vi "Populate Column Headers.vi"(8 "error in (no error)":errorcluster, 11 "Column Headers":string[](array[string])) -> (0 "error out":errorcluster)   [LabVIEW 2023, in "RFCalAndFixtureCharact.Common.lvlib"]
uses:
  RFCalAndFixtureCharact.Common.lvlib
  Type Definitions/Dictionary Operation.ctl
  <vilib>/Utility/error.llb/Trim Whitespace One-Sided.vi
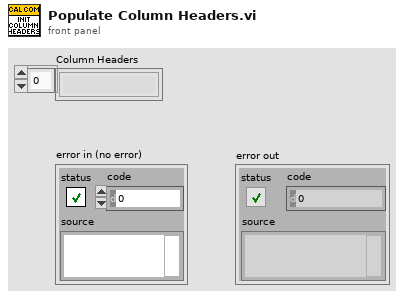
[diagram p1: front panel]
types:
  T1 = typedef "RFCalAndFixtureCharact.Common.lvlib/Dictionary Operation.ctl" = enum16{"Read", "Insert", "Remove", "Clear", "Get All", "Update"}
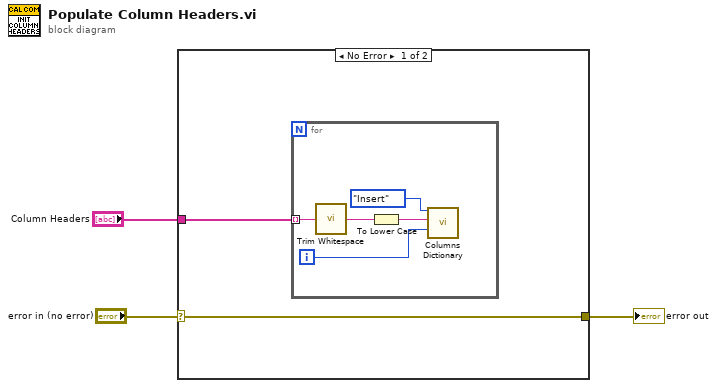
[diagram p0: block diagram]
diagram:
  n1 = case shown="No Error" "error in (no error)" {
    selector: "error in (no error)" -> [w5 w11]
    tunnel: [w5 w11] -> w2
    tunnel: "Column Headers" -> [w4 _]
    frame No Error {
      n2 = for {
        tunnel: w4 -> [w9] mode=indexing
        i -> [w8]
        n3 = call <vilib>:"Trim Whitespace.vi"("string"=w9) -> ("trimmed string"=w7:string)  [unwired: 1 in]
        n4 = To Lower Case(string=w7) -> (all lower case string=w6:string)
        n5 = call "Columns Dictionary.vi"("Action"=Dictionary_Operation."Insert", "Column Header"=w6, "Column Index"=w8) -> ()  [unwired: 10 in, 3 out]
      }
    }
    frame Error {
    }
  }
  "error out" <- w2
